vi "nominal asset attach dataset begin.vi"(8 "error in (no error)":errorcluster, 9 "out_staging":i32, 10 "dataset_rid":string, 11 "scope_name":string) -> (0 "error out":errorcluster, 1 "out_staging out":i32, 3 "function return":i32)   [LabVIEW 2020, in "client.lvlib"]
doc: "int32_t nominal_asset_attach_dataset_begin(const char *scope_name,\n const char *dataset_rid,\n int32_t *out_staging);"
uses:
  client.lvlib
  bin/nominalClient_64.dll
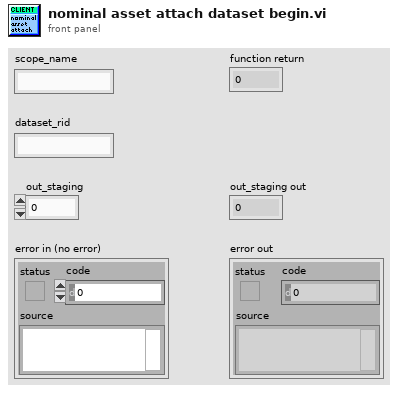
[diagram p1: front panel]
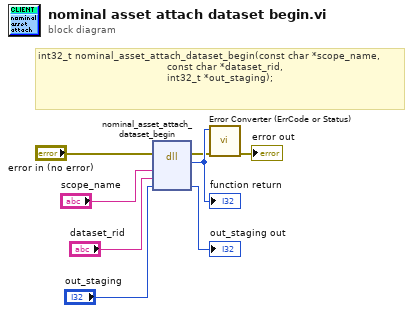
[diagram p0: block diagram]
diagram:
  # "int32_t nominal_asset_attach_dataset_begin(const char *scope_name,\n                                           const char *dataset_rid,\n                                           int32_t *out_staging);"
  n1 = dll-call lib="C:/code/labview-client-rs/lv_src/bin/nominalClient_*.*" fn="nominal_asset_attach_dataset_begin"(error in="error in (no error)", "scope_name"="scope_name", "dataset_rid"="dataset_rid", "out_staging"="out_staging") -> (error out=w2:errorcluster, w8:i32, "out_staging"=→"out_staging out":i32)  [unwired: 4 in, 1 out]
  "function return" <- w8
  n2 = call "Error Converter (ErrCode or Status).vi"("error in (no error)"=w2, "error code"=w8) -> ("error out"=→"error out":errorcluster)  [unwired: 9 in]
